vi "Append To Dataset 2D Integer.vi"(8 "error in (no error)":errorcluster, 9 "data":i32[][](array[numeric]), 11 "dataset_id":i32) -> (0 "error out":errorcluster, 3 "Dataset id out":i32)   [LabVIEW 2014]
uses:
  HDF5Tools.lvlib
  Release/HDF5Tools.dll
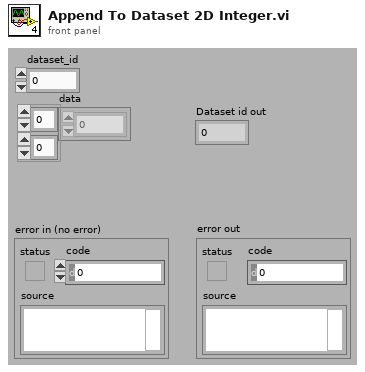
[diagram p1: front panel]
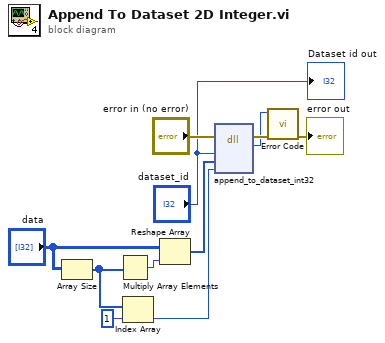
[diagram p0: block diagram]
diagram:
  n1 = Array Size(array="data") -> (size(s)=w7:i32[])
  n2 = Multiply Array Elements(1:w7) -> (0:w6:i32)
  n3 = Index Array(array=w7, index=1) -> (element=w4:i32)
  n4 = Reshape Array("data", w6) -> (w10:i32[])
  n5 = dll-call lib="C:/labview-acquisition/HDF5Tools32/Release/HDF5Tools.dll" fn="append_to_dataset_int32"(error in="error in (no error)", "dataset_id"="dataset_id", "data"=w10, "count"=w4) -> (error out=w2:errorcluster, "error"=w1:i32)  [unwired: 5 in, 1 out]
  n6 = call "Error Code.vi"("Error in"=w2, "Error code"=w1) -> ("Error out"=→"error out":errorcluster)  [unwired: 9 in]
  "Dataset id out" <- "dataset_id"
